vi "create.vi"(8 "error in (no error)":errorcluster, 10 "DetailedStates":T1=enum."StandbyState", 11 "StateFactory in":refnum<class "StateFactory.lvclass">) -> (0 "error out":errorcluster, 2 "State out":refnum<class "State.lvclass">, 3 "StateFactory out":refnum<class "StateFactory.lvclass">)   [LabVIEW 2016, in "StateFactory.lvclass"]
uses:
  StateFactory.lvclass
  DataTypes/Topics/Parts/DetailedStates.ctl
  State/State.lvclass
  OfflineState/OfflineState.lvclass
  D:/Code/ts_M1M3Support/States/State/State.lvclass
  InitialState/InitialState.lvclass
  StandbyState/StandbyState.lvclass
  DisabledState/DisabledState.lvclass
  ParkedState/ParkedState.lvclass
  FaultState/FaultState.lvclass
  ParkedMaintenanceState/ParkedMaintenanceState.lvclass
  ActiveMaintenanceState/ActiveMaintenanceState.lvclass
  DataTypes/Topics/M1M3SupportTopics.lvlib
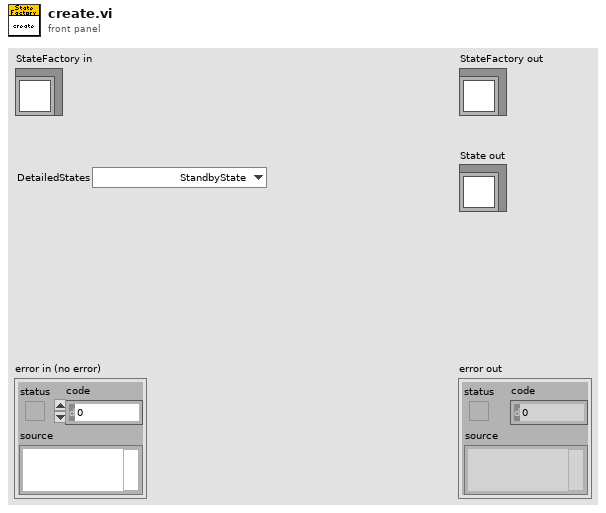
[diagram p1: front panel]
types:
  T1 = typedef "M1M3SupportTopics.lvlib/DetailedStates.ctl" = enum16{"OfflineState", "InitialState", "StandbyState", "DisabledState", "ParkedState", "FaultState", "ParkedMaintenanceState", "ActiveMaintenanceState"}
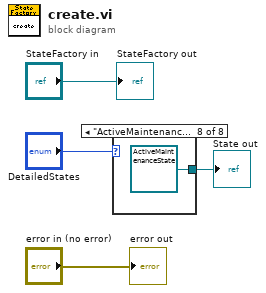
[diagram p0: block diagram]
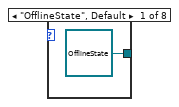
[diagram p2: hidden frame]
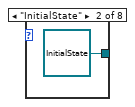
[diagram p3: hidden frame]
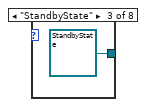
[diagram p4: hidden frame]
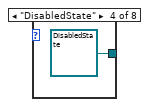
[diagram p5: hidden frame]
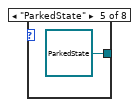
[diagram p6: hidden frame]
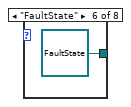
[diagram p7: hidden frame]
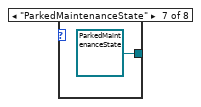
[diagram p8: hidden frame]
diagram:
  n1 = case shown="\"ActiveMaintenanceState\"" "DetailedStates" {
    tunnel: [refnum<class "OfflineState.lvclass"> refnum ("OfflineState.lvclass") refnum<class "InitialState.lvclass"> refnum ("InitialState.lvclass") refnum<class "StandbyState.lvclass"> refnum ("StandbyState.lvclass") refnum<class "DisabledState.lvclass"> refnum ("DisabledState.lvclass") refnum<class "ParkedState.lvclass"> refnum ("ParkedState.lvclass") refnum<class "FaultState.lvclass"> refnum ("FaultState.lvclass") refnum<class "ParkedMaintenanceState.lvclass"> refnum ("ParkedMaintenanceState.lvclass") refnum<class "ActiveMaintenanceState.lvclass"> refnum ("ActiveMaintenanceState.lvclass")] -> w1
    frame "OfflineState", Default {
    }
    frame "InitialState" {
    }
    frame "StandbyState" {
    }
    frame "DisabledState" {
    }
    frame "ParkedState" {
    }
    frame "FaultState" {
    }
    frame "ParkedMaintenanceState" {
    }
    frame "ActiveMaintenanceState" {
    }
  }
  "State out" <- w1
  "error out" <- "error in (no error)"
  "StateFactory out" <- "StateFactory in"
